vi "add.vi"(7 "waitgroup":T1, 8 "error in (no error)":errorcluster, 11 "timeout_ms":i32) -> (0 "error out":errorcluster)   [LabVIEW 2015, in "lv-waitgroup.lvlib"]
uses:
  lv-waitgroup.lvlib
  _controls/api_waitgroup.ctl
  _controls/data_error.ctl
  private/_controls/waitgroup.ctl
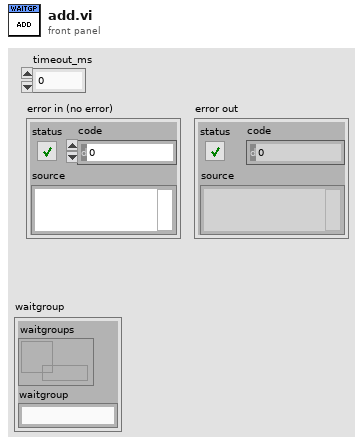
[diagram p1: front panel]
types:
  T1 = typedef "lv-waitgroup.lvlib/api_waitgroup.ctl" = cluster{"waitgroups":refnum<data-value>, "waitgroup":string}
  T2 = typedef "lv-waitgroup.lvlib/data_error.ctl" = enum16{"<data_error>", "unable_to_generate_id", "waitgroup_not_found", "unable_to_add_to_waitgroup", "<null>"}
  T3 = typedef "lv-waitgroup.lvlib/waitgroup.ctl" = cluster{"waitgroup":refnum<queue>, "queues":variant}
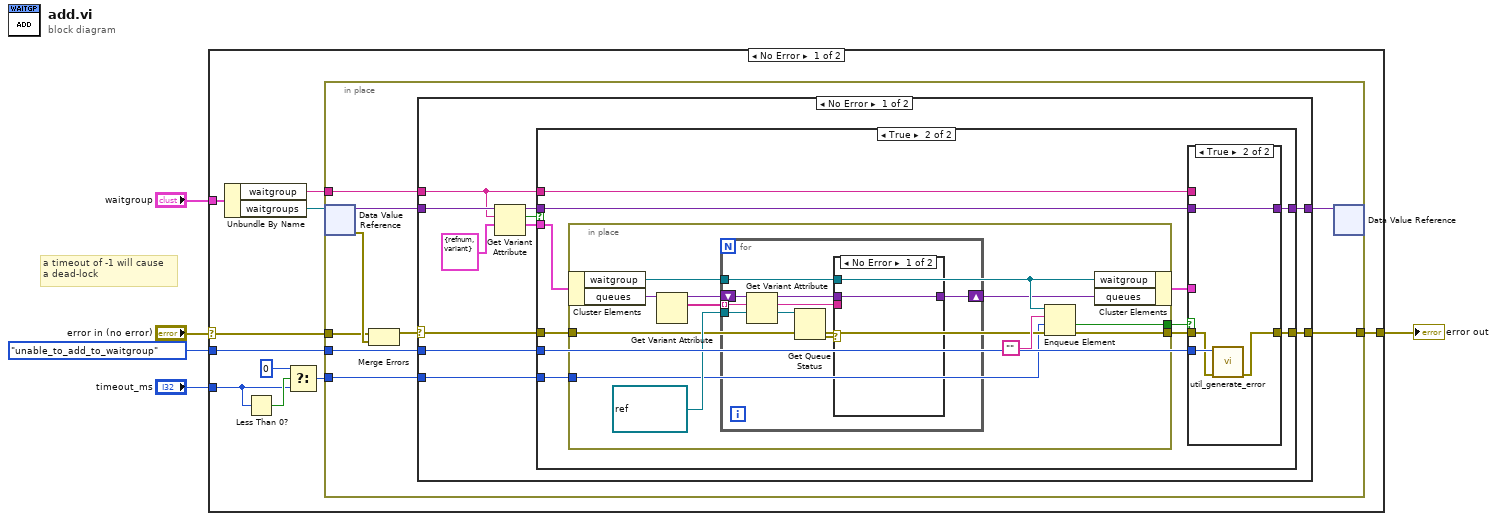
[diagram p0: block diagram]
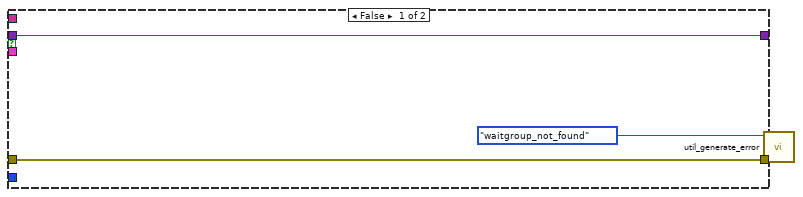
[diagram p2: hidden frame]
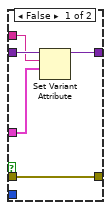
[diagram p3: hidden frame]
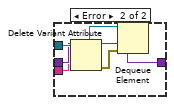
[diagram p4: hidden frame]
diagram:
  # "a timeout of -1 will cause\na dead-lock"
  n1 = case shown="No Error" "error in (no error)" {
    selector: "error in (no error)" -> [w6 w87]
    tunnel: [w15 w87] -> w4
    tunnel: "waitgroup" -> [w9 _]
    tunnel: data_error."unable_to_add_to_waitgroup" ("data_error") -> [w14 _]
    tunnel: "timeout_ms" -> [w12 _]
    frame No Error {
      n2 = Unbundle By Name(w9) -> ("waitgroup"=w8:string, "waitgroups"=w7:refnum<data-value>)
      n3 = Less Than 0?(x=w12) -> (x < 0?=w13:bool)
      n4 = Select(t=0, s=w13, f=w12) -> (s? t:f=w11:i32)
      n5 = in-place {
        in-place-border: [w24] -> w15
        in-place-border: w6 -> [w22]
        in-place-border: w8 -> [w19]
        in-place-border: w14 -> [w17]
        in-place-border: w11 -> [w16]
        n6 = in-place-dvr #1(w7) -> (w21:variant, w23:errorcluster)
        n7 = Merge Errors(w22, w23) -> (w18:errorcluster)
        n8 = case shown="No Error" w18 {
          selector: w18 -> [w28 w86]
          tunnel: [w35 w86] -> w24
          tunnel: w21 -> [w34 w85]
          tunnel: [w30 w85] -> w20
          tunnel: w19 -> [w29 _]
          tunnel: w17 -> [w26 _]
          tunnel: w16 -> [w25 _]
          frame No Error {
            n9 = Get Variant Attribute(Variant=w34, name=w29, default value (empty Variant)=T3 {"waitgroup"=refnum, "queues"=variant(refnum<queue>[] [])} ("shared_data")) -> (duplicate Variant=w32:variant, found=w27:bool, value=w31:T3)  [unwired: 1 in, 1 out]
            n10 = case shown="True" w27 {
              tunnel: [w36 w41] -> w35
              tunnel: w32 -> [w39 w50]
              tunnel: w31 -> [_ w49]
              tunnel: [w39 w48] -> w30
              tunnel: w29 -> [_ w46]
              tunnel: w28 -> [w37 w45]
              tunnel: w26 -> [_ w42]
              tunnel: w25 -> [_ w40]
              frame False {
                n11 = call "util_generate_error.vi"("error in (no error)"=w37, "data_error"=data_error."waitgroup_not_found") -> ("error out"=w36:errorcluster)  [unwired: 9 in]
              }
              frame True {
                n12 = in-place {
                  in-place-border: w45 -> [w61]
                  in-place-border: [w70] -> w43
                  in-place-border: [w69] -> w44
                  in-place-border: w40 -> [w60]
                  n13 = in-place-cluster #2(w49) -> ("waitgroup"=w63:refnum<queue>, "queues"=w67:variant)
                  n14 = Get Variant Attribute(Variant=w67) -> (duplicate Variant=w66:variant, names=w65:string[])  [unwired: 3 in, 2 out]
                  n15 = for {
                    tunnel: w65 -> [w72] mode=indexing
                    tunnel: refnum<queue> refnum ("queue") -> [w77]
                    tunnel: w63 -> [w73]
                    shift-right: [w71] -> w62
                    shift-left: w66 -> [w78]
                    n16 = Get Variant Attribute(Variant=w78, name=w72, default value (empty Variant)=w77) -> (duplicate Variant=w74:variant, value=w76:refnum<queue>)  [unwired: 1 in, 2 out]
                    n17 = Get Queue Status(queue=w76) -> (error out=w75:errorcluster)  [unwired: 2 in, 7 out]
                    n18 = case shown="No Error" w75 {
                      tunnel: w74 -> [w79 w83]
                      tunnel: w73 -> [_ w84]
                      tunnel: w72 -> [_ w82]
                      tunnel: [w79 w80] -> w71
                      frame No Error {
                      }
                      frame Error {
                        n19 = Delete Variant Attribute(6:w82, 7:w83) -> (0:w81:errorcluster, 3:w80:variant)  [unwired: 1 in, 1 out]
                        n20 = Dequeue Element(queue=w84, error in (no error)=w81) -> ()  [unwired: 1 in, 4 out]
                      }
                    }
                  }
                  n21 = Enqueue Element(queue=w63, element="", timeout in ms (-1)=w60, error in (no error)=w61) -> (timed out?=w69:bool, error out=w70:errorcluster)  [unwired: 1 out]
                  n22 = in-place-cluster #2("waitgroup"=w63, "queues"=w62) -> (w47:T3)
                }
                n23 = case shown="True" w44 {
                  tunnel: w50 -> [w54 w57]
                  tunnel: [w53 w57] -> w48
                  tunnel: w47 -> [w51 _]
                  tunnel: w46 -> [w52 _]
                  tunnel: w43 -> [w55 w58]
                  tunnel: w42 -> [_ w59]
                  tunnel: [w55 w56] -> w41
                  frame False {
                    n24 = Set Variant Attribute(Variant=w54, name=w52, value=w51) -> (Variant out=w53:variant)  [unwired: 1 in, 2 out]
                  }
                  frame True {
                    n25 = call "util_generate_error.vi"("error in (no error)"=w58, "data_error"=w59) -> ("error out"=w56:errorcluster)  [unwired: 9 in]
                  }
                }
              }
            }
          }
          frame Error {
          }
        }
        n26 = in-place-dvr #1(w20) -> ()  [unwired: 2 out]
      }
    }
    frame Error {
    }
  }
  "error out" <- w4
